vi "CAN.FG.vi"(7 "Action":T1, 8 "error in (no error)":errorcluster, 10 "Diagnostics Basic Configuraiton":T2={"Interface"="", "Baud Rate"=0, "Diagnostic Protocol"=enum."GMLAN", "Transport Protocol"=enum."ISO TP - Normal Mode", "Transmit ID"=0, "Receive ID"=0, "Transmit Extension"=0, "Receive Extension"=0, "Receive UUDT ID"=0, "Enable Stream"=TRUE, "VW TP Channel ID"=0, "Fill Frame"=TRUE, "Fill Byte"=255, "Termination"=FALSE, "LIN Cluster"="ADCS_LIN_database", "NAD"=1, "IO Mode"=0, "Max DLC"=8, "FD Baud Rate"=0, "Security"={"Source DLL Path"=path "", "Security Level"=1, "Target DLL Path"=path ""}} {"IO Mode" items=["CAN 2.0", "CAN FD", "CAN FD+BRS"]; "Fill Byte" format="%.0x"; "VW TP Channel ID" format="%.0x"; "Receive UUDT ID" format="%.0x"; "Receive Extension" format="%.0x"; "Transmit Extension" format="%.0x"; "Receive ID" format="%.0x"; "Transmit ID" format="%.0x"}, 11 "Device Item Ref in":T7 format="%.0x") -> (0 "error out":errorcluster, 2 "Diagnostics Basic Configuraiton":T2={"Interface"="", "Baud Rate"=0, "Diagnostic Protocol"=enum."GMLAN", "Transport Protocol"=enum."ISO TP - Normal Mode", "Transmit ID"=0, "Receive ID"=0, "Transmit Extension"=0, "Receive Extension"=0, "Receive UUDT ID"=0, "Enable Stream"=TRUE, "VW TP Channel ID"=0, "Fill Frame"=FALSE, "Fill Byte"=255, "Termination"=FALSE, "LIN Cluster"="ADCS_LIN_database", "NAD"=1, "IO Mode"=0, "Max DLC"=8, "FD Baud Rate"=0, "Security"={"Source DLL Path"=path "", "Security Level"=1, "Target DLL Path"=path ""}} {"IO Mode" items=["CAN 2.0", "CAN FD", "CAN FD+BRS"]; "Fill Byte" format="%.0x"; "VW TP Channel ID" format="%.0x"; "Receive UUDT ID" format="%.0x"; "Receive Extension" format="%.0x"; "Transmit Extension" format="%.0x"; "Receive ID" format="%.0x"; "Transmit ID" format="%.0x"}, 3 "Device Item Ref out":T7=18446744073709551615 format="%.0x")   [LabVIEW 2015, in "Diagnostics Addon System Explorer.lvlib"]
uses:
  Diagnostics Addon System Explorer.lvlib
  <vilib>/NI Veristand/Custom Device API/Custom Device Item Ref.ctl
  Shared/Types/CAN.ctl
  Shared/Types/CAN.Interface.ctl
  Shared/Types/Protocol.ctl
  Shared/Types/Transport.ctl
  Shared/Types/Security.ctl
  Types/FG.Action.ctl
  <vilib>/NI/NI VeriStand Advanced SysDef API/_SubVIs/SysDef.Property.Set.U32.vi
  <vilib>/NI/NI VeriStand Advanced SysDef API/_SubVIs/SysDef.Property.Set.String.vi
  <vilib>/NI/NI VeriStand Advanced SysDef API/_SubVIs/SysDef.Property.Set.Boolean.vi
  <vilib>/NI/NI VeriStand Advanced SysDef API/SysDef API/SysDef.Property.Remove.vi
  <vilib>/NI/NI VeriStand Advanced SysDef API/_SubVIs/SysDef.Property.Set.DependentFile.vi
  <vilib>/Utility/MD5Checksum.llb/MD5Checksum File.vi
  Shared/SubVIs/Constants.vi
  <vilib>/NI Veristand/Custom Device API/Get Item Property (U32).vi
  <vilib>/NI Veristand/Custom Device API/Get Item Property (String).vi
  <vilib>/NI Veristand/Custom Device API/Get Item Property (Boolean).vi
  Shared/Diagnostics Addon Shared.lvlib
  <vilib>/NI VeriStand/Custom Device API/Custom Device API.lvlib
  <vilib>/NI/NI VeriStand Advanced SysDef API/SysDef API/Advanced System Definition.lvlib
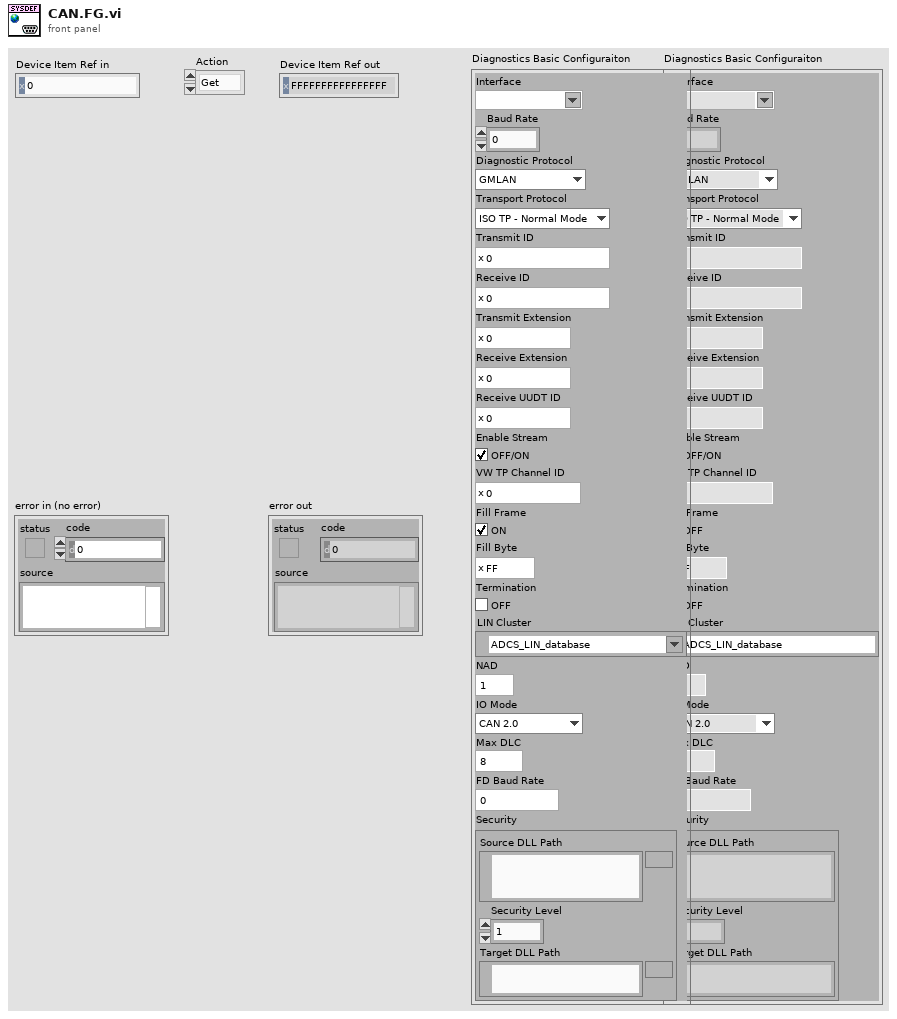
[diagram p1: front panel]
types:
  T1 = typedef "Diagnostics Addon System Explorer.lvlib/FG.Action.ctl" = enum16{"Get", "Set"}
  T2 = typedef "Diagnostics Addon Shared.lvlib/CAN.ctl" = cluster{"Interface":T3, "Baud Rate":u32, "Diagnostic Protocol":T4, "Transport Protocol":T5, "Transmit ID":u32, "Receive ID":u32, "Transmit Extension":u8, "Receive Extension":u8, "Receive UUDT ID":u32, "Enable Stream":bool, "VW TP Channel ID":u32, "Fill Frame":bool, "Fill Byte":u8, "Termination":bool, "LIN Cluster":refnum<k21>, "NAD":u8, "IO Mode":u32, "Max DLC":u16, "FD Baud Rate":u32, "Security":T6}
  T3 = typedef "Diagnostics Addon Shared.lvlib/CAN.Interface.ctl" = string
  T4 = typedef "Diagnostics Addon Shared.lvlib/Protocol.ctl" = enum16{"GMLAN", "KWP-2000", "UDS", "User-Defined"}
  T5 = typedef "Diagnostics Addon Shared.lvlib/Transport.ctl" = enum16{"ISO TP - Normal Mode", "ISO TP - Mixed Mode", "VW TP 2.0", "Diagnostics on IP", "ISO TP LIN"}
  T6 = typedef "Diagnostics Addon Shared.lvlib/Security.ctl" = cluster{"Source DLL Path":path, "Security Level":u8, "Target DLL Path":path}
  T7 = typedef "Custom Device API.lvlib/Custom Device Item Ref.ctl" = u64
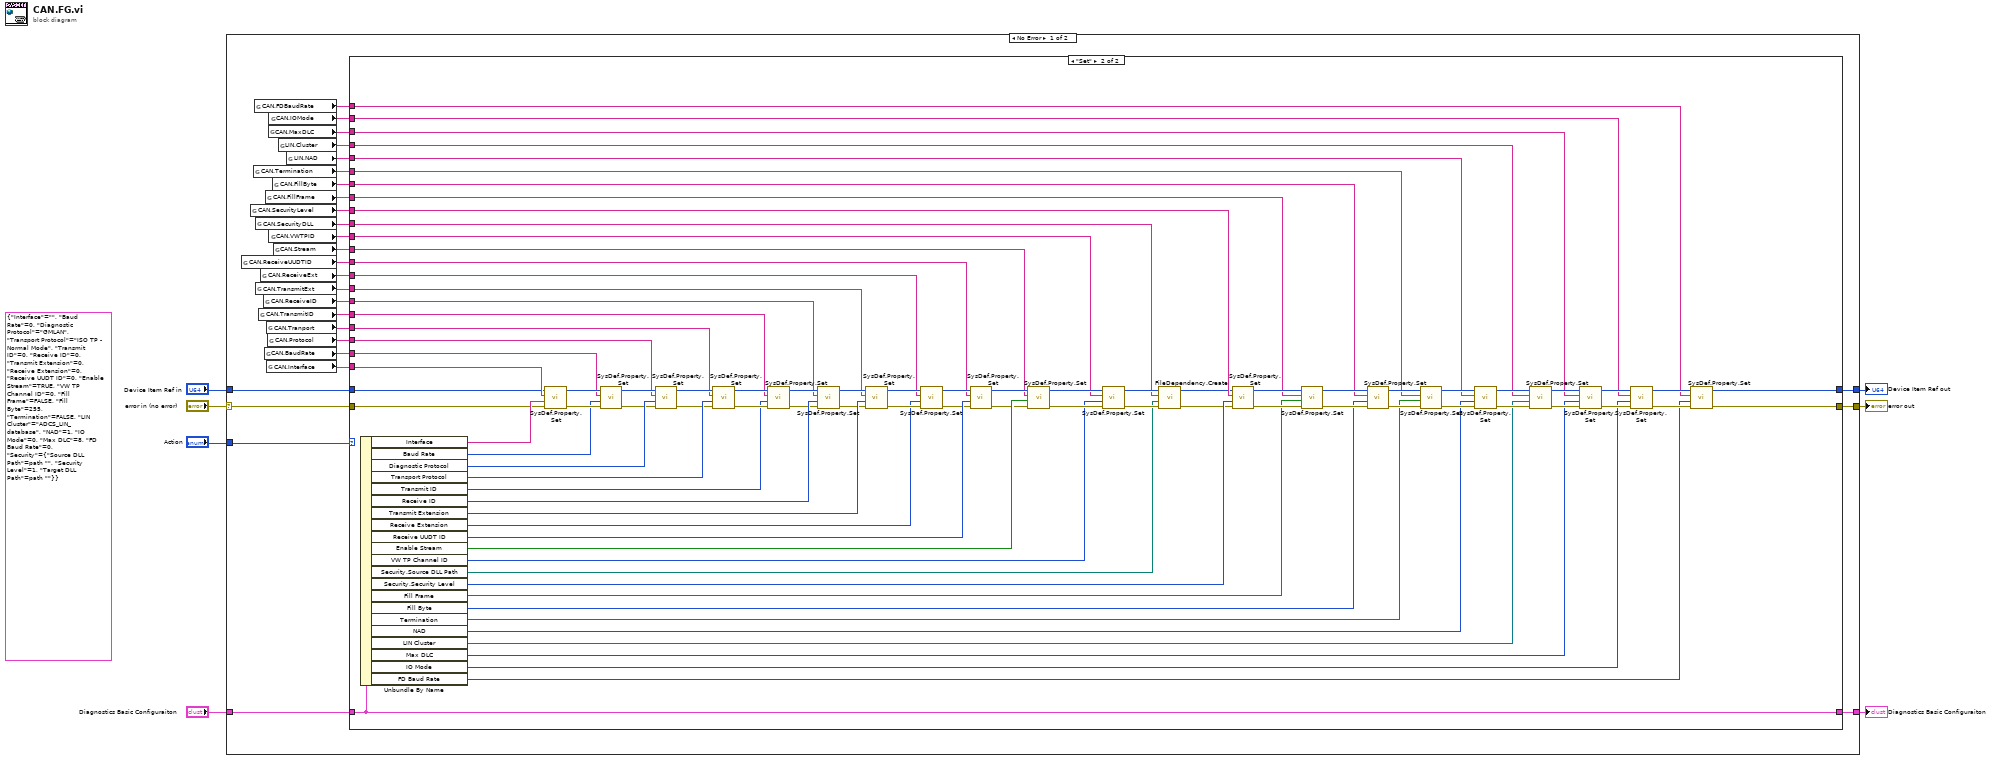
[diagram p0: block diagram]
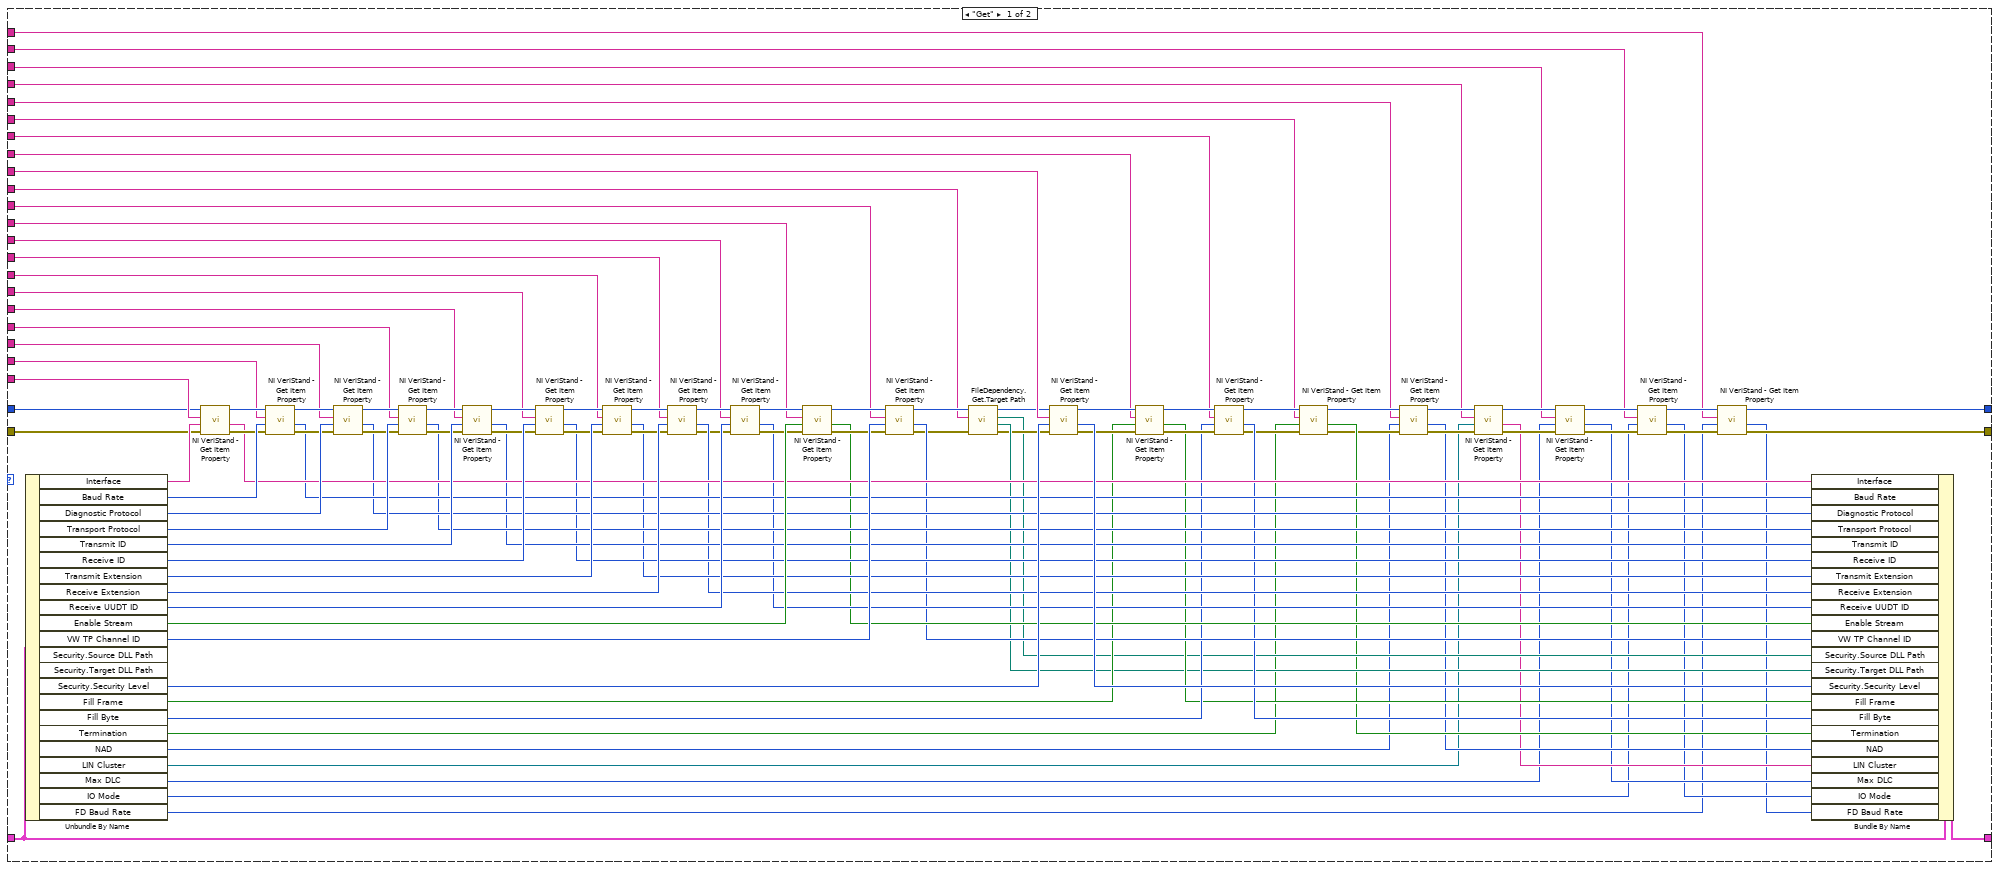
[diagram p2: hidden frame]
diagram:
  (unwired) T2 {"Interface"="", "Baud Rate"=0, "Diagnostic Protocol"=enum."GMLAN", "Transport Protocol"=enum."ISO TP - Normal Mode", "Transmit ID"=0, "Receive ID"=0, "Transmit Extension"=0, "Receive Extension"=0, "Receive UUDT ID"=0, "Enable Stream"=TRUE, "VW TP Channel ID"=0, "Fill Frame"=FALSE, "Fill Byte"=255, "Termination"=FALSE, "LIN Cluster"="ADCS_LIN_database", "NAD"=1, "IO Mode"=0, "Max DLC"=8, "FD Baud Rate"=0, "Security"={"Source DLL Path"=path "", "Security Level"=1, "Target DLL Path"=path ""}} ("Diagnostics Basic Configuraiton 2")
  n1 = case shown="No Error" "error in (no error)" {
    selector: "error in (no error)" -> [w35 w232]
    tunnel: "Device Item Ref in" -> [w34 w233]
    tunnel: [w33 w233] -> w4
    tunnel: [w32 w232] -> w5
    tunnel: [w31 _] -> w3
    tunnel: "Diagnostics Basic Configuraiton" -> [w30 _]
    tunnel: "Action" -> [w29 _]
    frame No Error {
      n2 = global read "Constants.vi" "CAN.ReceiveUUDTID"() -> (w20:string)
      n3 = global read "Constants.vi" "CAN.SecurityLevel"() -> (w16:string)
      n4 = global read "Constants.vi" "CAN.Termination"() -> (w13:string)
      n5 = global read "Constants.vi" "CAN.FDBaudRate"() -> (w12:string)
      n6 = global read "Constants.vi" "CAN.SecurityDLL"() -> (w17:string)
      n7 = global read "Constants.vi" "CAN.TransmitExt"() -> (w22:string)
      n8 = global read "Constants.vi" "CAN.TransmitID"() -> (w24:string)
      n9 = global read "Constants.vi" "CAN.ReceiveExt"() -> (w21:string)
      n10 = global read "Constants.vi" "CAN.ReceiveID"() -> (w23:string)
      n11 = global read "Constants.vi" "CAN.BaudRate"() -> (w27:string)
      n12 = global read "Constants.vi" "CAN.FillFrame"() -> (w15:string)
      n13 = global read "Constants.vi" "CAN.Tranport"() -> (w25:string)
      n14 = global read "Constants.vi" "CAN.Interface"() -> (w28:string)
      n15 = global read "Constants.vi" "CAN.Protocol"() -> (w26:string)
      n16 = global read "Constants.vi" "CAN.MaxDLC"() -> (w10:string)
      n17 = global read "Constants.vi" "CAN.IOMode"() -> (w11:string)
      n18 = global read "Constants.vi" "CAN.VWTPID"() -> (w18:string)
      n19 = global read "Constants.vi" "CAN.FillByte"() -> (w14:string)
      n20 = global read "Constants.vi" "CAN.Stream"() -> (w19:string)
      n21 = global read "Constants.vi" "LIN.Cluster"() -> (w9:string)
      n22 = global read "Constants.vi" "LIN.NAD"() -> (w8:string)
      n23 = case shown="\"Set\"" w29 {
        tunnel: w35 -> [w64 w168]
        tunnel: w34 -> [w63 w167]
        tunnel: [w55 w157] -> w33
        tunnel: [w57 w158] -> w32
        tunnel: [w143 w231] -> w31
        tunnel: w30 -> [w144 w231]
        tunnel: w28 -> [w98 w198]
        tunnel: w27 -> [w97 w197]
        tunnel: w26 -> [w96 w196]
        tunnel: w25 -> [w95 w195]
        tunnel: w24 -> [w94 w194]
        tunnel: w23 -> [w93 w193]
        tunnel: w22 -> [w92 w192]
        tunnel: w21 -> [w91 w191]
        tunnel: w20 -> [w90 w190]
        tunnel: w19 -> [w89 w189]
        tunnel: w18 -> [w88 w188]
        tunnel: w17 -> [w74 w174]
        tunnel: w16 -> [w87 w187]
        tunnel: w15 -> [w78 w176]
        tunnel: w14 -> [w77 w177]
        tunnel: w13 -> [w65 w170]
        tunnel: w8 -> [w50 w149]
        tunnel: w9 -> [w49 w148]
        tunnel: w10 -> [w48 w147]
        tunnel: w11 -> [w47 w146]
        tunnel: w12 -> [w46 w145]
        frame "Get" {
          n24 = Unbundle By Name(w144) -> ("Interface"=w142:T3, "Baud Rate"=w141:u32, "Diagnostic Protocol"=w140:T4, "Transport Protocol"=w139:T5, "Transmit ID"=w138:u32, "Receive ID"=w137:u32, "Transmit Extension"=w136:u8, "Receive Extension"=w135:u8, "Receive UUDT ID"=w134:u32, "Enable Stream"=w133:bool, "VW TP Channel ID"=w132:u32, "Security.Security Level"=w131:u8, "Fill Frame"=w82:bool, "Fill Byte"=w81:u8, "Termination"=w67:bool, "NAD"=w45:u8, "LIN Cluster"=w43:refnum<k21>, "Max DLC"=w38:u16, "IO Mode"=w37:u32, "FD Baud Rate"=w36:u32)  [unwired: 2 out]
          n25 = call-poly <vilib>:"NI VeriStand - Get Item Property.vi"("error in (no error)"=w64, "Default Value"=w142, "Property Name"=w98, "Item Ref in"=w63) -> ("error out"=w112:errorcluster, "Value"=w110:string, "Item Ref out"=w130:T7)  [unwired: 4 in, 1 out]
          n26 = call-poly <vilib>:"NI VeriStand - Get Item Property.vi"("error in (no error)"=w112, "Default Value"=w141, "Property Name"=w97, "Item Ref in"=w130) -> ("error out"=w113:errorcluster, "Value"=w109:u32, "Item Ref out"=w129:T7)  [unwired: 4 in, 1 out]
          n27 = call-poly <vilib>:"NI VeriStand - Get Item Property.vi"("error in (no error)"=w113, "Default Value"=w140, "Property Name"=w96, "Item Ref in"=w129) -> ("error out"=w114:errorcluster, "Value"=w108:u32, "Item Ref out"=w128:T7)  [unwired: 4 in, 1 out]
          n28 = call-poly <vilib>:"NI VeriStand - Get Item Property.vi"("error in (no error)"=w114, "Default Value"=w139, "Property Name"=w95, "Item Ref in"=w128) -> ("error out"=w115:errorcluster, "Value"=w107:u32, "Item Ref out"=w127:T7)  [unwired: 4 in, 1 out]
          n29 = call-poly <vilib>:"NI VeriStand - Get Item Property.vi"("error in (no error)"=w115, "Default Value"=w138, "Property Name"=w94, "Item Ref in"=w127) -> ("error out"=w116:errorcluster, "Value"=w106:u32, "Item Ref out"=w126:T7)  [unwired: 4 in, 1 out]
          n30 = call-poly <vilib>:"NI VeriStand - Get Item Property.vi"("error in (no error)"=w116, "Default Value"=w137, "Property Name"=w93, "Item Ref in"=w126) -> ("error out"=w117:errorcluster, "Value"=w105:u32, "Item Ref out"=w125:T7)  [unwired: 4 in, 1 out]
          n31 = call-poly <vilib>:"NI VeriStand - Get Item Property.vi"("error in (no error)"=w117, "Default Value"=w136, "Property Name"=w92, "Item Ref in"=w125) -> ("error out"=w118:errorcluster, "Value"=w104:u32, "Item Ref out"=w124:T7)  [unwired: 4 in, 1 out]
          n32 = call-poly <vilib>:"NI VeriStand - Get Item Property.vi"("error in (no error)"=w118, "Default Value"=w135, "Property Name"=w91, "Item Ref in"=w124) -> ("error out"=w102:errorcluster, "Value"=w103:u32, "Item Ref out"=w123:T7)  [unwired: 4 in, 1 out]
          n33 = call-poly <vilib>:"NI VeriStand - Get Item Property.vi"("error in (no error)"=w102, "Default Value"=w134, "Property Name"=w90, "Item Ref in"=w123) -> ("error out"=w119:errorcluster, "Value"=w101:u32, "Item Ref out"=w122:T7)  [unwired: 4 in, 1 out]
          n34 = call-poly <vilib>:"NI VeriStand - Get Item Property.vi"("error in (no error)"=w119, "Default Value"=w133, "Property Name"=w89, "Item Ref in"=w122) -> ("error out"=w120:errorcluster, "Value"=w100:bool, "Item Ref out"=w121:T7)  [unwired: 4 in, 1 out]
          n35 = call-poly <vilib>:"NI VeriStand - Get Item Property.vi"("error in (no error)"=w120, "Default Value"=w132, "Property Name"=w88, "Item Ref in"=w121) -> ("error out"=w75:errorcluster, "Value"=w99:u32, "Item Ref out"=w76:T7)  [unwired: 4 in, 1 out]
          n36 = call "FileDependency.Get.Target Path.vi"("error in (no error)"=w75, "Bitfile 986x"=w74, "Item Ref in"=w76) -> ("error out"=w72:errorcluster, "Target Path"=w73:path, "Source Path"=w70:path, "Item Ref out"=w71:T7)  [unwired: 5 in]
          n37 = call-poly <vilib>:"NI VeriStand - Get Item Property.vi"("error in (no error)"=w72, "Default Value"=w131, "Property Name"=w87, "Item Ref in"=w71) -> ("error out"=w84:errorcluster, "Value"=w111:u32, "Item Ref out"=w83:T7)  [unwired: 4 in, 1 out]
          n38 = call-poly <vilib>:"NI VeriStand - Get Item Property.vi"("error in (no error)"=w84, "Default Value"=w82, "Property Name"=w78, "Item Ref in"=w83) -> ("error out"=w86:errorcluster, "Value"=w79:bool, "Item Ref out"=w85:T7)  [unwired: 4 in, 1 out]
          n39 = call-poly <vilib>:"NI VeriStand - Get Item Property.vi"("error in (no error)"=w86, "Default Value"=w81, "Property Name"=w77, "Item Ref in"=w85) -> ("error out"=w68:errorcluster, "Value"=w80:u32, "Item Ref out"=w69:T7)  [unwired: 4 in, 1 out]
          n40 = call-poly <vilib>:"NI VeriStand - Get Item Property.vi"("error in (no error)"=w68, "Default Value"=w67, "Property Name"=w65, "Item Ref in"=w69) -> ("error out"=w58:errorcluster, "Value"=w66:bool, "Item Ref out"=w54:T7)  [unwired: 4 in, 1 out]
          n41 = call-poly <vilib>:"NI VeriStand - Get Item Property.vi"("error in (no error)"=w58, "Default Value"=w45, "Property Name"=w50, "Item Ref in"=w54) -> ("error out"=w62:errorcluster, "Value"=w44:u32, "Item Ref out"=w53:T7)  [unwired: 4 in, 1 out]
          n42 = call-poly <vilib>:"NI VeriStand - Get Item Property.vi"("error in (no error)"=w62, "Default Value"=w43, "Property Name"=w49, "Item Ref in"=w53) -> ("error out"=w61:errorcluster, "Value"=w42:string, "Item Ref out"=w52:T7)  [unwired: 4 in, 1 out]
          n43 = call-poly <vilib>:"NI VeriStand - Get Item Property.vi"("error in (no error)"=w61, "Default Value"=w38, "Property Name"=w48, "Item Ref in"=w52) -> ("error out"=w60:errorcluster, "Value"=w41:u32, "Item Ref out"=w51:T7)  [unwired: 4 in, 1 out]
          n44 = call-poly <vilib>:"NI VeriStand - Get Item Property.vi"("error in (no error)"=w60, "Default Value"=w37, "Property Name"=w47, "Item Ref in"=w51) -> ("error out"=w59:errorcluster, "Value"=w40:u32, "Item Ref out"=w56:T7)  [unwired: 4 in, 1 out]
          n45 = call-poly <vilib>:"NI VeriStand - Get Item Property.vi"("error in (no error)"=w59, "Default Value"=w36, "Property Name"=w46, "Item Ref in"=w56) -> ("error out"=w57:errorcluster, "Value"=w39:u32, "Item Ref out"=w55:T7)  [unwired: 4 in, 1 out]
          n46 = Bundle By Name(cluster=w144, "Interface"=w110, "Baud Rate"=w109, "Diagnostic Protocol"=w108, "Transport Protocol"=w107, "Transmit ID"=w106, "Receive ID"=w105, "Transmit Extension"=w104, "Receive Extension"=w103, "Receive UUDT ID"=w101, "Enable Stream"=w100, "VW TP Channel ID"=w99, "Security.Source DLL Path"=w70, "Security.Target DLL Path"=w73, "Security.Security Level"=w111, "Fill Frame"=w79, "Fill Byte"=w80, "Termination"=w66, "NAD"=w44, "LIN Cluster"=w42, "Max DLC"=w41, "IO Mode"=w40, "FD Baud Rate"=w39) -> (w143:T2)
        }
        frame "Set" {
          n47 = Unbundle By Name(w231) -> ("Interface"=w230:T3, "Baud Rate"=w227:u32, "Diagnostic Protocol"=w220:T4, "Transport Protocol"=w219:T5, "Transmit ID"=w218:u32, "Receive ID"=w217:u32, "Transmit Extension"=w216:u8, "Receive Extension"=w215:u8, "Receive UUDT ID"=w214:u32, "Enable Stream"=w213:bool, "VW TP Channel ID"=w212:u32, "Security.Source DLL Path"=w173:path, "Security.Security Level"=w211:u8, "Fill Frame"=w179:bool, "Fill Byte"=w178:u8, "Termination"=w169:bool, "NAD"=w154:u8, "LIN Cluster"=w153:refnum<k21>, "Max DLC"=w152:u16, "IO Mode"=w151:u32, "FD Baud Rate"=w150:u32)
          n48 = call-poly <vilib>:"SysDef.Property.Set.vi"("error in (no error)"=w168, "Value"=w230, "Property Name"=w198, "nodeID"=w167) -> ("error out"=w228:errorcluster, "nodeID out"=w229:u64)  [unwired: 6 in]
          n49 = call-poly <vilib>:"SysDef.Property.Set.vi"("error in (no error)"=w228, "Value"=w227, "Property Name"=w197, "nodeID"=w229) -> ("error out"=w199:errorcluster, "nodeID out"=w210:u64)  [unwired: 6 in]
          n50 = call-poly <vilib>:"SysDef.Property.Set.vi"("error in (no error)"=w199, "Value"=w220, "Property Name"=w196, "nodeID"=w210) -> ("error out"=w200:errorcluster, "nodeID out"=w209:u64)  [unwired: 6 in]
          n51 = call-poly <vilib>:"SysDef.Property.Set.vi"("error in (no error)"=w200, "Value"=w219, "Property Name"=w195, "nodeID"=w209) -> ("error out"=w226:errorcluster, "nodeID out"=w225:u64)  [unwired: 6 in]
          n52 = call-poly <vilib>:"SysDef.Property.Set.vi"("error in (no error)"=w226, "Value"=w218, "Property Name"=w194, "nodeID"=w225) -> ("error out"=w201:errorcluster, "nodeID out"=w208:u64)  [unwired: 6 in]
          n53 = call-poly <vilib>:"SysDef.Property.Set.vi"("error in (no error)"=w201, "Value"=w217, "Property Name"=w193, "nodeID"=w208) -> ("error out"=w202:errorcluster, "nodeID out"=w207:u64)  [unwired: 6 in]
          n54 = call-poly <vilib>:"SysDef.Property.Set.vi"("error in (no error)"=w202, "Value"=w216, "Property Name"=w192, "nodeID"=w207) -> ("error out"=w222:errorcluster, "nodeID out"=w221:u64)  [unwired: 6 in]
          n55 = call-poly <vilib>:"SysDef.Property.Set.vi"("error in (no error)"=w222, "Value"=w215, "Property Name"=w191, "nodeID"=w221) -> ("error out"=w203:errorcluster, "nodeID out"=w206:u64)  [unwired: 6 in]
          n56 = call-poly <vilib>:"SysDef.Property.Set.vi"("error in (no error)"=w203, "Value"=w214, "Property Name"=w190, "nodeID"=w206) -> ("error out"=w204:errorcluster, "nodeID out"=w205:u64)  [unwired: 6 in]
          n57 = call-poly <vilib>:"SysDef.Property.Set.vi"("error in (no error)"=w204, "Value"=w213, "Property Name"=w189, "nodeID"=w205) -> ("error out"=w223:errorcluster, "nodeID out"=w224:u64)  [unwired: 6 in]
          n58 = call-poly <vilib>:"SysDef.Property.Set.vi"("error in (no error)"=w223, "Value"=w212, "Property Name"=w188, "nodeID"=w224) -> ("error out"=w182:errorcluster, "nodeID out"=w175:u64)  [unwired: 6 in]
          n59 = call "FileDependency.Create.vi"("error in (no error)"=w182, "DLL Path"=w173, "DLL Property Name"=w174, "Item Ref in"=w175) -> ("error out"=w181:errorcluster, "Item Ref out"=w180:T7)  [unwired: 6 in]
          n60 = call-poly <vilib>:"SysDef.Property.Set.vi"("error in (no error)"=w181, "Value"=w211, "Property Name"=w187, "nodeID"=w180) -> ("error out"=w185:errorcluster, "nodeID out"=w183:u64)  [unwired: 6 in]
          n61 = call-poly <vilib>:"SysDef.Property.Set.vi"("error in (no error)"=w185, "Value"=w179, "Property Name"=w176, "nodeID"=w183) -> ("error out"=w186:errorcluster, "nodeID out"=w184:u64)  [unwired: 6 in]
          n62 = call-poly <vilib>:"SysDef.Property.Set.vi"("error in (no error)"=w186, "Value"=w178, "Property Name"=w177, "nodeID"=w184) -> ("error out"=w172:errorcluster, "nodeID out"=w171:u64)  [unwired: 6 in]
          n63 = call-poly <vilib>:"SysDef.Property.Set.vi"("error in (no error)"=w172, "Value"=w169, "Property Name"=w170, "nodeID"=w171) -> ("error out"=w166:errorcluster, "nodeID out"=w165:u64)  [unwired: 6 in]
          n64 = call-poly <vilib>:"SysDef.Property.Set.vi"("error in (no error)"=w166, "Value"=w154, "Property Name"=w149, "nodeID"=w165) -> ("error out"=w164:errorcluster, "nodeID out"=w163:u64)  [unwired: 6 in]
          n65 = call-poly <vilib>:"SysDef.Property.Set.vi"("error in (no error)"=w164, "Value"=w153, "Property Name"=w148, "nodeID"=w163) -> ("error out"=w161:errorcluster, "nodeID out"=w162:u64)  [unwired: 6 in]
          n66 = call-poly <vilib>:"SysDef.Property.Set.vi"("error in (no error)"=w161, "Value"=w152, "Property Name"=w147, "nodeID"=w162) -> ("error out"=w155:errorcluster, "nodeID out"=w160:u64)  [unwired: 6 in]
          n67 = call-poly <vilib>:"SysDef.Property.Set.vi"("error in (no error)"=w155, "Value"=w151, "Property Name"=w146, "nodeID"=w160) -> ("error out"=w156:errorcluster, "nodeID out"=w159:u64)  [unwired: 6 in]
          n68 = call-poly <vilib>:"SysDef.Property.Set.vi"("error in (no error)"=w156, "Value"=w150, "Property Name"=w145, "nodeID"=w159) -> ("error out"=w158:errorcluster, "nodeID out"=w157:u64)  [unwired: 6 in]
        }
      }
    }
    frame Error {
    }
  }
  "error out" <- w5
  "Device Item Ref out" <- w4
  "Diagnostics Basic Configuraiton" <- w3
